vi "Multi_Calib_Prog.vi"() -> ()   [LabVIEW 2021]
uses:
  Anemometry Sub Vis/Calibration/Calib_mode.ctl
  Anemometry Sub Vis/Controls/User_Specific_mode.ctl
  Anemometry Sub Vis/Controls/Setup.ctl
  Anemometry Sub Vis/Controls/Post_Process.ctl
  Anemometry Sub Vis/Controls/Save_Data.ctl
  Anemometry Sub Vis/Globals/Meas_global.vi
panel:
  out "Calibration Filenames":path[](array[path])
  in  "Files Selected":bool
  in  "Select Calib Files":i32[](listbox)
  in  "Mode":T1(ring)
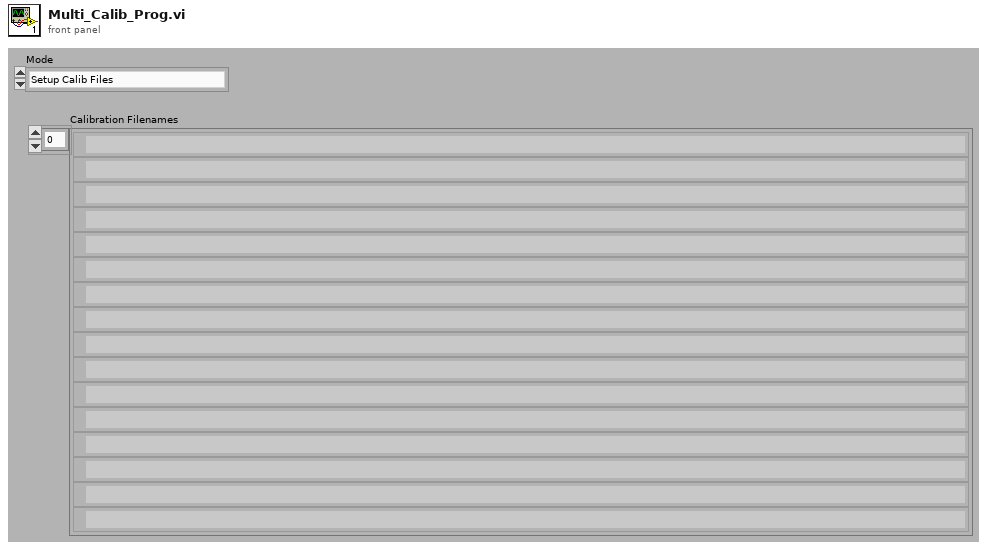
[diagram p1: front panel]
types:
  T1 = enum16{"Setup Calib Files", "Add New Point to Calib Files"}
  T2 = typedef "User_Specific_mode.ctl" = enum16{"Check VI only", "Run VI"}
  T3 = typedef "Calib_mode.ctl" = enum16{"Show Setup", "Take a New Calibration Point", "Refit Curve", "Setup Front Panel"}
  T4 = typedef "Save_Data.ctl" = enum16{"Save No Data", "Save Data"}
  T5 = typedef "Post_Process.ctl" = enum16{"Take New Data", "Post Process Raw Data File"}
  T6 = typedef "Setup.ctl" = enum16{"Run Program", "Show Setup", "Save Current Setup", "Setup Front Panel"}
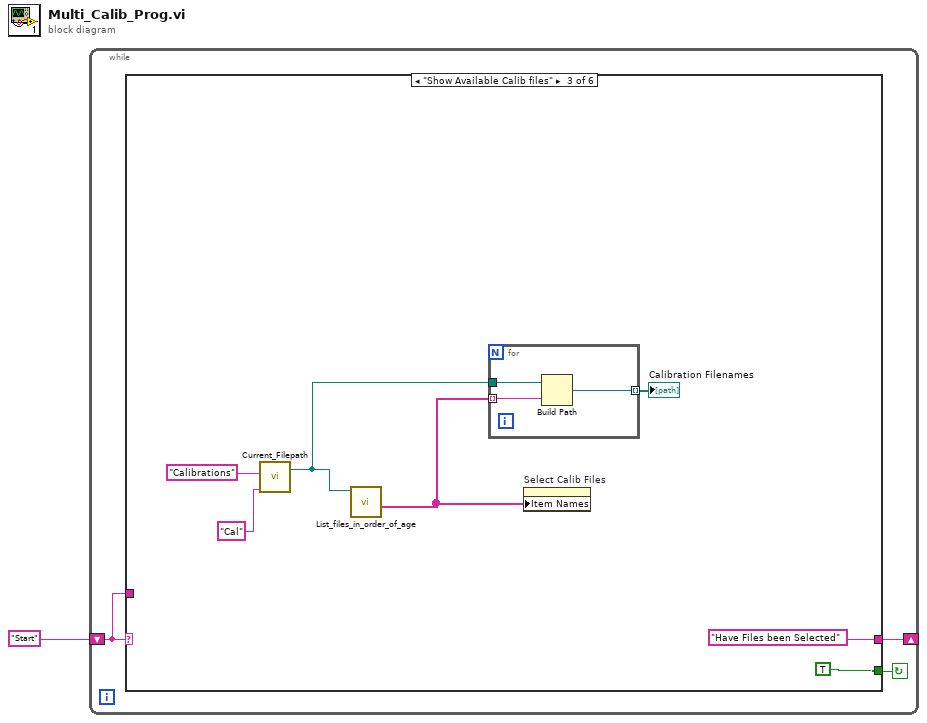
[diagram p0: block diagram]
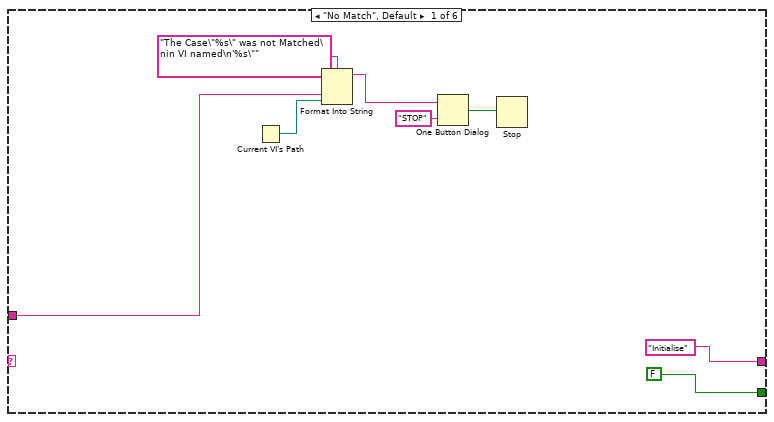
[diagram p2: hidden frame]
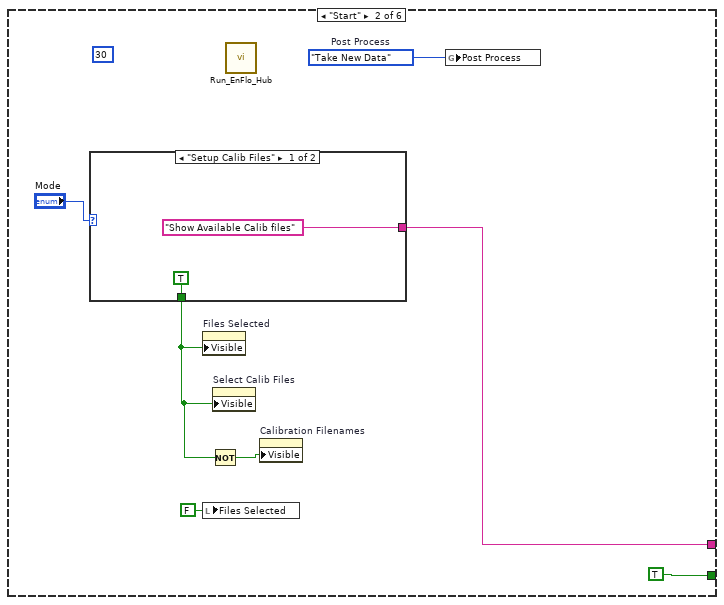
[diagram p3: hidden frame]
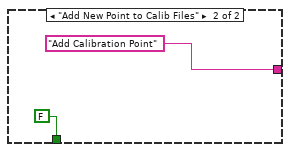
[diagram p4: hidden frame]
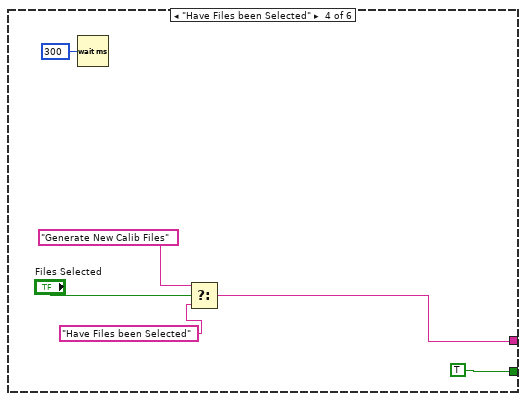
[diagram p5: hidden frame]
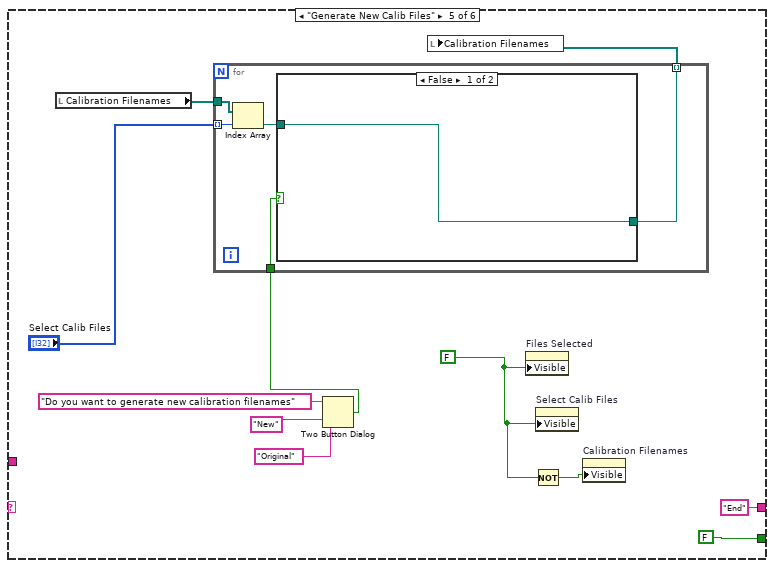
[diagram p6: hidden frame]
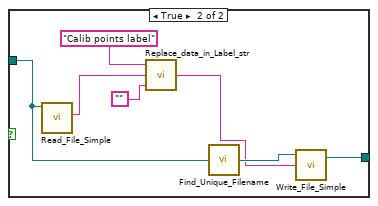
[diagram p7: hidden frame]
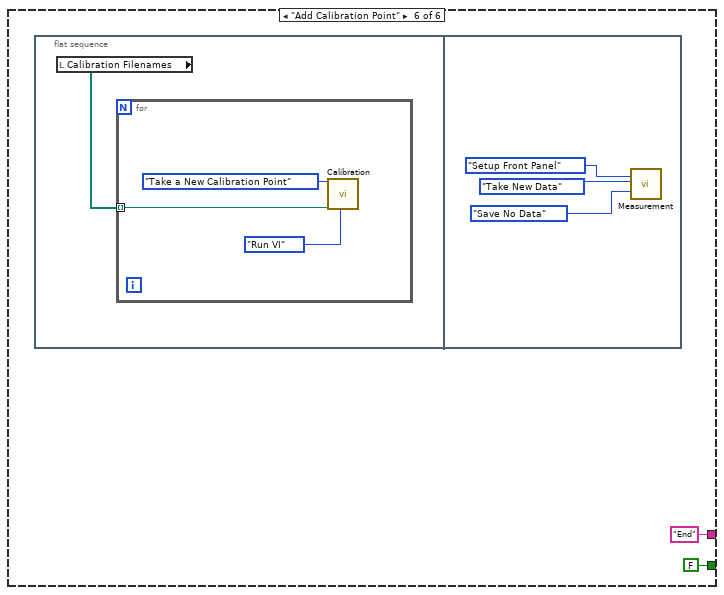
[diagram p8: hidden frame]
diagram:
  n1 = while {
    shift-left: "Start" -> [w2]
    shift-right: [w3] -> _
    stop <- w4 continue-if-true
    n2 = case shown="\"Show Available Calib files\"" w2 {
      tunnel: [FALSE TRUE TRUE TRUE FALSE FALSE] -> w4
      tunnel: ["Initialise" w17 "Have Files been Selected" w36 "End" ("t") "End" ("t")] -> w3
      tunnel: w2 -> [w7 _ _ _ _ _]
      frame "No Match", Default {
        n3 = Current VI's Path() -> (path=w6:path)
        n4 = Format Into String(format string="The Case\"%s\" was not Matched\nin VI named\n'%s\"" ("Format String"), w7, w6) -> (resulting string=w10:string)  [unwired: 2 in, 1 out]
        n5 = One Button Dialog(message=w10, button name ("OK")="STOP") -> (true=w8:bool)
        n6 = Stop(stop? (T)=w8) -> ()
      }
      frame "Start" {
        (unwired) 30
        w13 = Post_Process."Take New Data"  # Post Process
        n7 = case shown="\"Setup Calib Files\"" "Mode" {
          tunnel: ["Show Available Calib files" "Add Calibration Point"] -> w17
          tunnel: [TRUE FALSE] -> w15
          frame "Setup Calib Files" {
          }
          frame "Add New Point to Calib Files" {
          }
        }
        n8 = property on="Files Selected" class="Bool (strict)"("Visible"=w15) -> ()  [unwired: 2 in, 2 out]
        n9 = local write "Files Selected"(FALSE ("Files Selected")) -> ()
        n10 = Not(x=w15) -> (.not. x?=w14:bool)
        n11 = property on="Select Calib Files" class="LstBox (strict)"("Visible"=w15) -> ()  [unwired: 2 in, 2 out]
        n12 = call "Run_EnFlo_Hub.vi"() -> ()  [unwired: 7 in, 1 out]
        n13 = property on="Calibration Filenames" class="Arr (strict)"("Visible"=w14) -> ()  [unwired: 2 in, 2 out]
        n14 = global write "Meas_global.vi" "Post Process"(w13) -> ()
      }
      frame "Show Available Calib files" {
        n15 = call "Current_Filepath.vi"("Short_Name"="Cal" ("Data Type"), "Data Type"="Calibrations") -> ("Directory"=w26:path)  [unwired: 2 in, 1 out]
        n16 = call "List_files_in_order_of_age.vi"("Folder"=w26) -> ("file names"=w25:string[])  [unwired: 10 in]
        n17 = for {
          tunnel: w26 -> [w33]
          tunnel: w25 -> [w32] mode=indexing
          tunnel: [w31] -> w27 mode=indexing
          n18 = Build Path(base path=w33, name or relative path=w32) -> (appended path=w31:path)
        }
        "Calibration Filenames" <- w27
        n19 = property on="Select Calib Files" class="LstBox (strict)"("Item Names"=w25) -> ()  [unwired: 2 in, 2 out]
      }
      frame "Have Files been Selected" {
        n20 = Wait (ms)(milliseconds to wait=u32 300) -> ()  [unwired: 1 out]
        n21 = Select(t="Generate New Calib Files", s="Files Selected", f="Have Files been Selected") -> (s? t:f=w36:string)
      }
      frame "Generate New Calib Files" {
        w44 = FALSE ("Visible")
        n22 = local read "Calibration Filenames"() -> (w49:path[])
        n23 = Two Button Dialog(message="Do you want to generate new calibration filenames", 1:"Original" ("F button name (\"Cancel\")"), 2:"New" ("T button name (\"OK\")")) -> (T button?=w40:bool)
        n24 = for {
          tunnel: w49 -> [w55]
          tunnel: "Select Calib Files" -> [w54] mode=indexing
          tunnel: [w52] -> w47 mode=indexing
          tunnel: w40 -> [w51]
          n25 = Index Array(array=w55, index=w54) -> (element=w53:path)
          n26 = case shown="False" w51 {
            tunnel: w53 -> [w56 w60]
            tunnel: [w56 w57] -> w52
            frame False {
            }
            frame True {
              n27 = call "Read_File_Simple.vi"("Filename"=w60) -> ("string"=w62:string)  [unwired: 4 in, 5 out]
              n28 = call "Replace_data_in_Label_str.vi"("New data string"="", "Input string"=w62, "Variable name"="Calib points label") -> ("Appended string"=w58:string)
              n29 = call "Find_Unique_Filename.vi"("Path In"=w60) -> ("Unique Path Out"=w59:path)  [unwired: 2 in]
              n30 = call "Write_File_Simple.vi"("character string"=w58, "file path"=w59) -> ("file path Out"=w57:path)  [unwired: 1 in, 1 out]
            }
          }
        }
        n31 = local write "Calibration Filenames"(w47) -> ()
        n32 = property on="Files Selected" class="Bool (strict)"("Visible"=w44) -> ()  [unwired: 2 in, 2 out]
        n33 = Not(x=w44) -> (.not. x?=w45:bool)
        n34 = property on="Select Calib Files" class="LstBox (strict)"("Visible"=w44) -> ()  [unwired: 2 in, 2 out]
        n35 = property on="Calibration Filenames" class="Arr (strict)"("Visible"=w45) -> ()  [unwired: 2 in, 2 out]
      }
      frame "Add Calibration Point" {
        n36 = flat-sequence {
          frame #0 {
            n37 = local read "Calibration Filenames"() -> (w66:path[])
            n38 = for {
              tunnel: w66 -> [w68] mode=indexing
              n39 = call "Calibration.vi"("Mode"=Calib_mode."Take a New Calibration Point", "Calib file"=w68, "Simulate/Run"=User_Specific_mode."Run VI") -> ()  [unwired: 14 in, 3 out]
            }
          }
          frame #1 {
            n40 = call "Measurement.vi"("setup"=Setup."Setup Front Panel", "Post Process"=Post_Process."Take New Data", "File"=Save_Data."Save No Data") -> ()  [unwired: 3 in, 14 out]
          }
        }
      }
    }
  }
